vi "Create Flags.vi"(8 "error in":errorcluster, 9 "Color":T1[](array[typedef])=[enum."Red", enum."Blue", enum."Green", enum."Yellow"], 10 "State":bool[](array[boolean])=[FALSE, FALSE, FALSE, FALSE], 11 "Room Number":u8) -> (0 "error out":errorcluster, 3 "reference out":refnum<class "Flags.lvclass">)   [LabVIEW 2015, in "Flags.lvclass"]
uses:
  Flags.lvclass
  ColorEnum.ctl
  Flags.lvclass/Flags.ctl
  Write Color.vi
  Write State.vi
  Write Room Number.vi
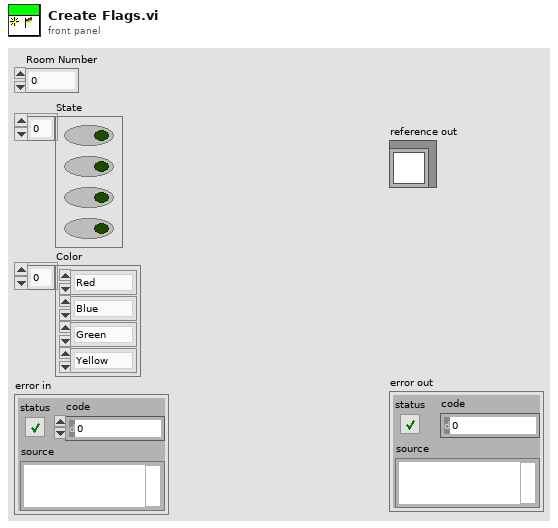
[diagram p1: front panel]
types:
  T1 = typedef "Flags.lvclass/ColorEnum.ctl" = enum8{"Red", "Blue", "Green", "Yellow"}
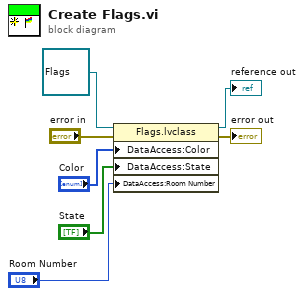
[diagram p0: block diagram]
diagram:
  n1 = property class="Flags.lvclass"(reference=refnum<class "Flags.lvclass"> refnum ("Flags.lvclass"), error in="error in", "DataAccess:Color"="Color", "DataAccess:State"="State", "DataAccess:Room Number"="Room Number") -> (reference out=→"reference out":refnum<class "Flags.lvclass">, error out=→"error out":errorcluster)
